vi "创建数据库.vi"(11 "路径 i":path=path "D:/MyAccessDB.mdb" caption="ACCESS数据库MDB文件") -> (0 "错误输出":errorcluster, 3 "路径 o":path=path "D:/MyAccessDB.mdb" caption="ACCESS数据库MDB文件")   [LabVIEW 2013]
panel:
  in  "ADOX._Catalog":refnum<k7>
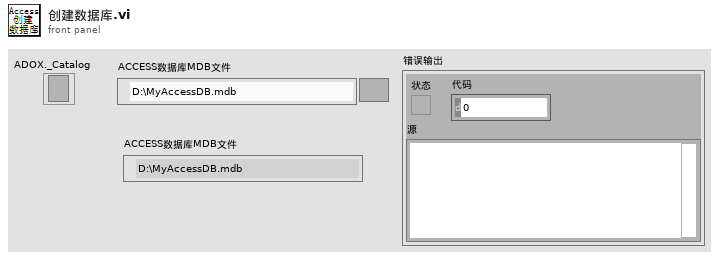
[diagram p1: front panel]
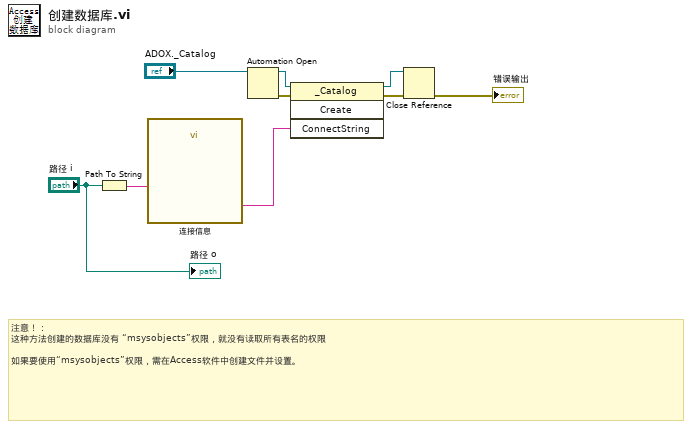
[diagram p0: block diagram]
diagram:
  # "注意！：\n这种方法创建的数据库没有 “msysobjects”权限，就没有读取所有表名的权限\n\n如果要使用“msysobjects”权限，需在Access软件中创建文件并设置。"
  n1 = Path To String(path="路径 i") -> (string=w4:string)
  n2 = call "连接信息"("文件路径"=w4) -> ("Result"=w3:string)  [unwired: 13 in, 1 out]
  n3 = Automation Open ("打开自动化")(Automation Refnum="ADOX._Catalog") -> (Automation Refnum=w6:refnum<k7>, error out=w7:errorcluster)  [unwired: 3 in]
  n4 = invoke class="_Catalog" method="Create"(reference=w6, error in=w7, "ConnectString"=w3) -> (reference out=w1:refnum<k7>, error out=w8:errorcluster)  [unwired: 1 in, 2 out]
  n5 = Close Reference(reference=w1, error in (no error)=w8) -> (error out=→"错误输出":errorcluster)
  "路径 o" <- "路径 i"
